vi "spiAccelerometerReadByte.vi"(2 "error in (no error)":errorcluster, 3 "Address":u8, 4 "Multiple bytes":bool) -> (0 "error out":errorcluster, 1 "Data":u16)   [LabVIEW 2012]
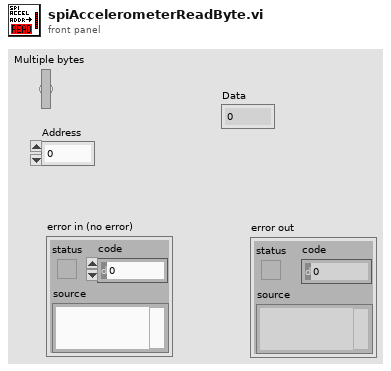
[diagram p1: front panel]
types:
  T1 = typedef "WPI_SPIDevRef.ctl" = cluster{"DevStatus":errorcluster}
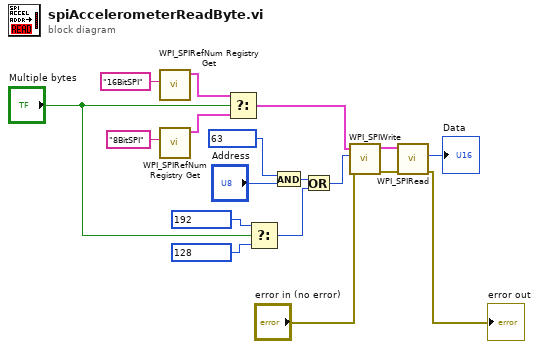
[diagram p0: block diagram]
diagram:
  n1 = call <vilib>:"WPI_SPIRefNum Registry Get.vi"("refnum name"="16BitSPI") -> ("SPIDevRef"=w11:T1)  [unwired: 9 in, 1 out]
  n2 = call <vilib>:"WPI_SPIRefNum Registry Get.vi"("refnum name"="8BitSPI") -> ("SPIDevRef"=w10:T1)  [unwired: 9 in, 1 out]
  n3 = Select(t=w11, s="Multiple bytes", f=w10) -> (s? t:f=w9:T1)
  n4 = Select(t=u8 192, s="Multiple bytes", f=u8 128) -> (s? t:f=w5:u8)
  n5 = And(x=u8 63, y="Address") -> (x .and. y?=w4:u8)
  n6 = Or(x=w4, y=w5) -> (x .or. y?=w15:u8)
  n7 = call <vilib>:"WPI_SPIWrite.vi"("error in (no error)"="error in (no error)", "Data To Send"=w15, "SPIDevRef"=w9) -> ("error out"=w17:errorcluster, "SPIDevRef"=w18:T1)  [unwired: 7 in]
  n8 = call <vilib>:"WPI_SPIRead.vi"("error in (no error)"=w17, "SPIDevRef"=w18) -> ("error out"=→"error out":errorcluster, "Received Data"=→"Data":u32)  [unwired: 7 in, 1 out]
